vi "DLLfinder.vi"() -> (1 "File Path":path)   [LabVIEW 2022 SP3]
panel:
  # "Provides  path to appropriate DLL for platform bitness"
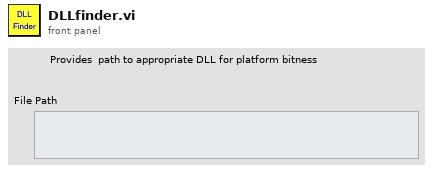
[diagram p1: front panel]
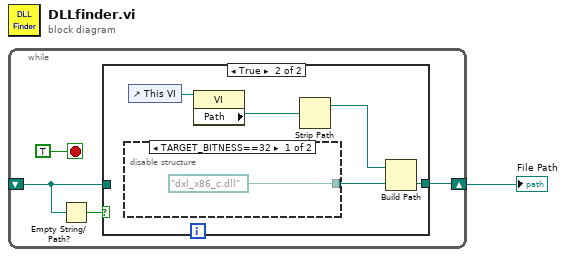
[diagram p0: block diagram]
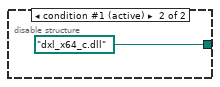
[diagram p3: hidden frame]
diagram:
  n1 = while {
    shift-right: [w2] -> w1
    shift-left: _ -> [w3]
    stop <- TRUE stop-if-true
    n2 = Empty String/Path?(string/path=w3) -> (empty?=w4:bool)
    n3 = case shown="True" w4 {
      tunnel: w3 -> [w6 _]
      tunnel: [w6 w8] -> w2
      frame False {
      }
      frame True {
        n4 = disable-structure shown="TARGET_BITNESS==32" {
          disable-tunnel: [path "dxl_x86_c.dll" path "dxl_x64_c.dll"] -> w11
          frame condition #0 {
          }
          frame condition #1 (active) {
          }
        }
        n5 = control-ref of="This VI"() -> (w10:refnum<vi>)
        n6 = property class="VI"(reference=w10) -> ("Path"=w9:path)  [unwired: 1 in, 2 out]
        n7 = Strip Path(path=w9) -> (stripped path=w7:path)  [unwired: 1 out]
        n8 = Build Path(base path=w7, name or relative path=w11) -> (appended path=w8:path)
      }
    }
  }
  "File Path" <- w1
